vi "KlingerV2 Control.vi"(7 "Axe":u8(ring)=3 items=["W", "X", "Y", "Z"], 8 "error in":errorcluster, 9 "PosDem":dbl caption="Allez à" min=-79999.999 max=79999.999 step=0.001 format="%.3f", 10 "Relatif":bool caption="Relatif/Absolu\n(Absolu)", 11 "VISA Rsrc":refnum<visa-resource-name>="SR530") -> (0 "error out":errorcluster, 1 "Position":dbl min=-79999.999 max=79999.999 step=0.001 format="%.3f", 2 "NLimit":bool caption="Limite -", 3 "PLimit":bool caption="Limite +", 5 "Axe out":u8(ring)=3 caption="Axe" items=["W", "X", "Y", "Z"])   [LabVIEW 2019]
doc: "Ce Vi est une interface de contrôle complète d'où on peut effectué les diverse fonction du contrôlleur Klinger"
uses:
  <vilib>/Utility/error.llb/DialogType.ctl
  <userlib>/KlingerV2/KlingerV2 Params.ctl
  <userlib>/KlingerV2/KlingerV2 ConvUnitArr.vi
panel:
  in  "Save Par":bool
  in  "WriteAcc":bool
  in  "WriteSpeed":bool
  in  "Enable":bool caption="Motor\nEnable"
  in  "ReadPos":bool
  in  "ModParam":bool
  out "Nom de l'axe":string
  out "CorrParams":T1={"CorrActive"=FALSE, "ErreurLim"=0.1, "NbrEssais"=3} caption="Paramètres de \ncorrection de position" {"NbrEssais" min=1 max=5 step=1; "ErreurLim" min=0.0 max=10.0 step=0.1 format="%#.1f"}
  in  "Unit":u8(ring) caption="Unité:" items=["Pas", "mm", "ps", "Degré (°)"]
  in  "Default":bool
  in  "Zero":bool
  in  "Accel":dbl=0.4000000059604645 caption="Accélération" min=0.10000000149011612 max=2.0 step=0.10000000149011612 format="%#.1f"
  in  "Speed Type":enum32{"Pas/Seconde", "ms/Pas"}(radio)
  in  "Vitesse":i32=800 min=32 max=4000 step=1 format="%#.0f"
  in  "Quitter":bool
  in  "RAZ":bool
  in  "Origine":bool
  out "PosErreur":dbl caption="Erreur de\nPositionnement" min=-79999.999 max=79999.999 step=0.001 format="%.3f"
  out "Indcomm":string caption="Terminal Indicateur"
  out "Pos Init":dbl caption="Position Initiale" min=-79999.999 max=79999.999 step=0.001 format="%.3f"
  out "Moving":bool caption="Déplacement\nen cours"
  out "Erreur":bool
  # "Commandes"
  # "Paramètres"
  # "Sec"
  # "Relatif"
  # "Absolu"
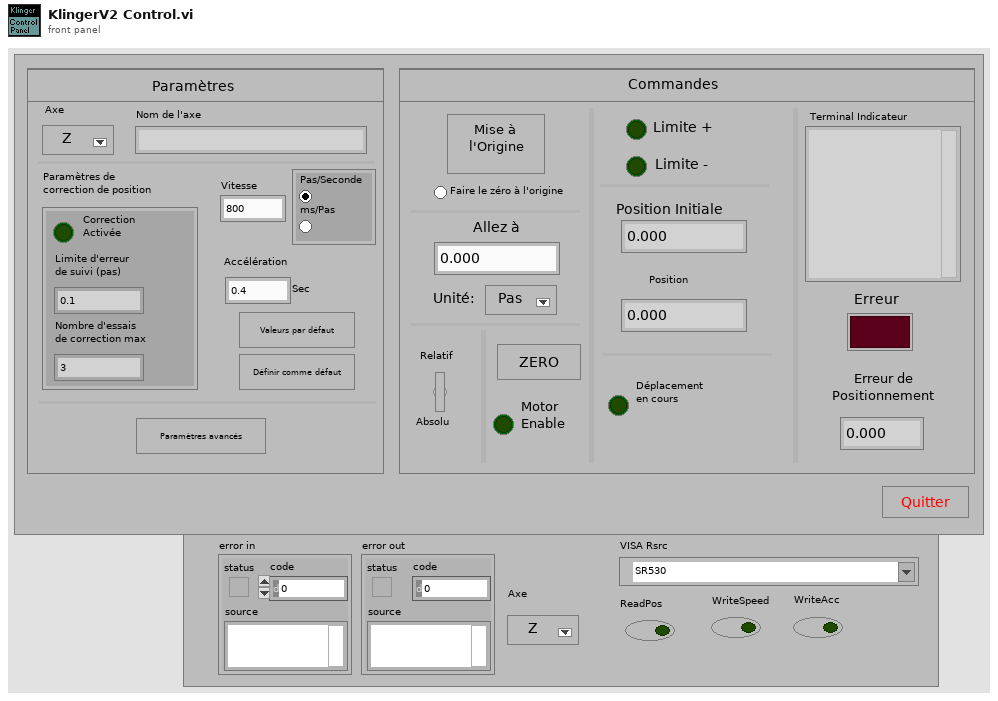
[diagram p1: front panel]
types:
  T1 = cluster{"CorrActive":bool, "ErreurLim":dbl, "NbrEssais":i32}
  T2 = cluster{"Position Ref":refnum<vi>, "Moving Ref":refnum<vi>, "PLimRef":refnum<vi>, "NLimRef":refnum<vi>}
  T3 = typedef "KlingerV2 Params.ctl" = enum16{"Type", "Origine", "Encodeur", "TypeMouv", "FactConv", "Nom", "CorrParams", "KlingCtrlPar", "Speed", "Acc", "Avance", "Tous"}
  T4 = cluster{"Minimum":dbl, "Maximum":dbl, "Increment":dbl}
  T5 = typedef "DialogType.ctl" = u16
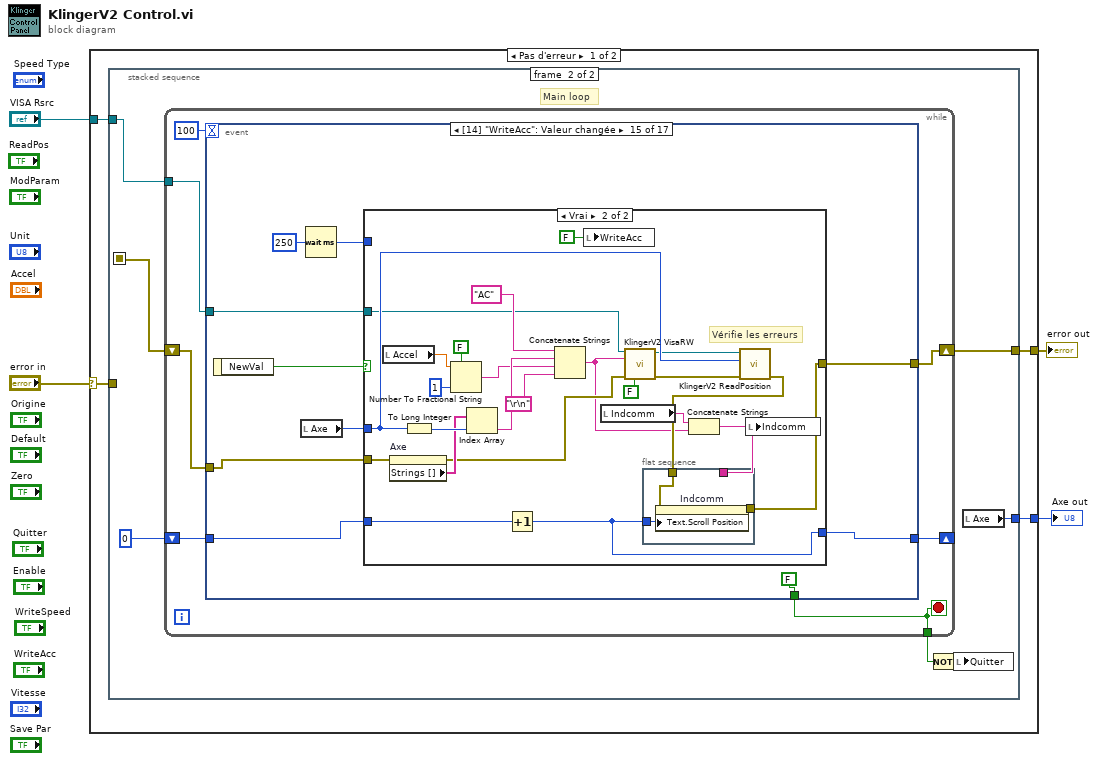
[diagram p0: block diagram]
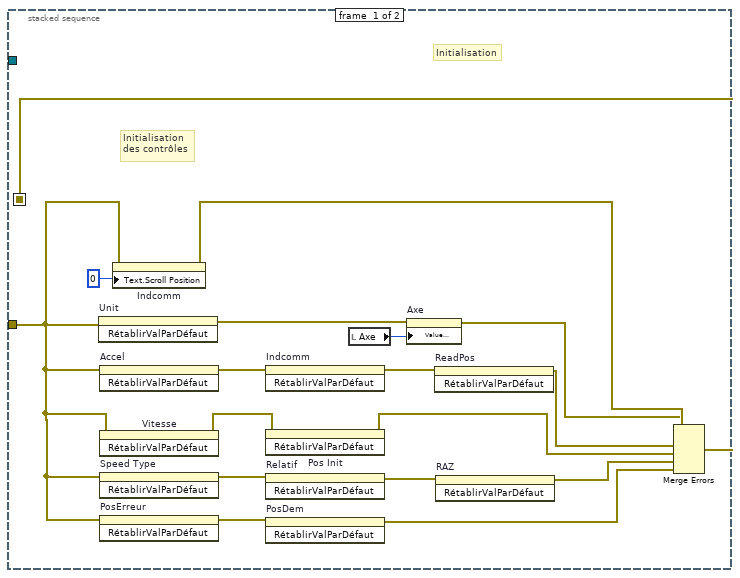
[diagram p2: hidden frame]
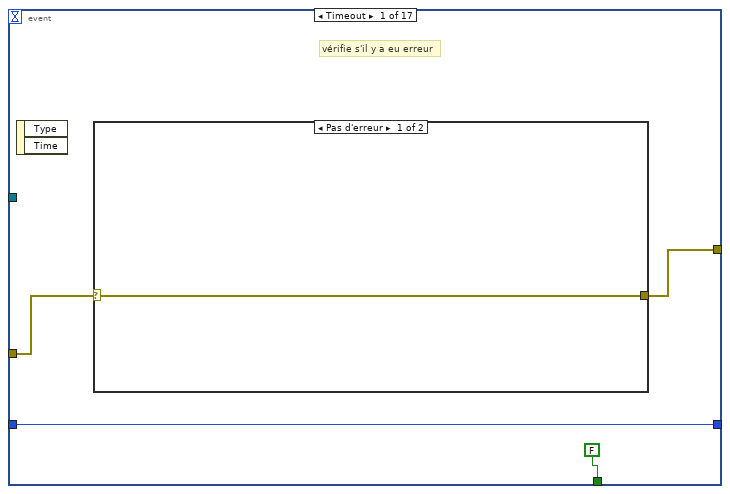
[diagram p3: hidden frame]
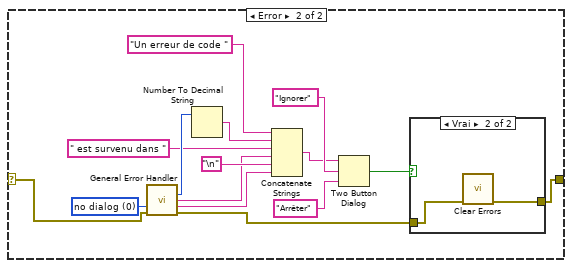
[diagram p4: hidden frame]
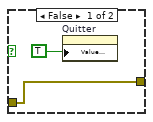
[diagram p5: hidden frame]
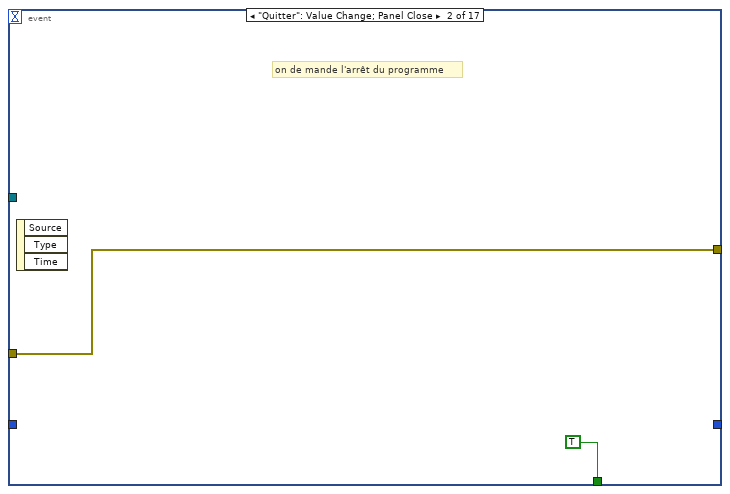
[diagram p6: hidden frame]
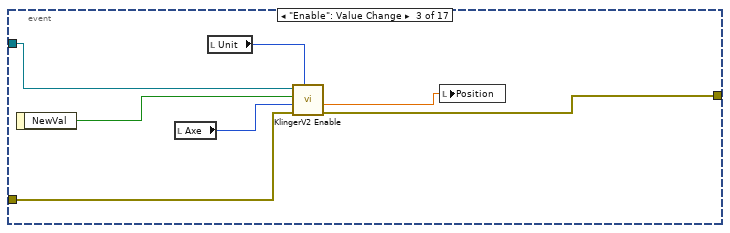
[diagram p7: hidden frame]
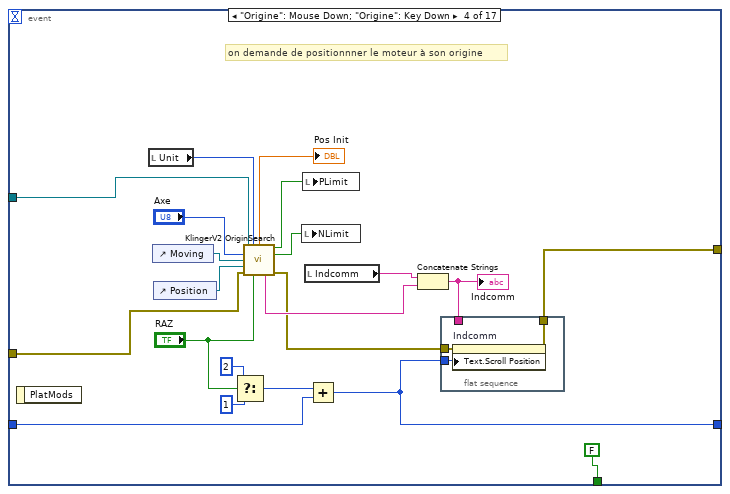
[diagram p8: hidden frame]
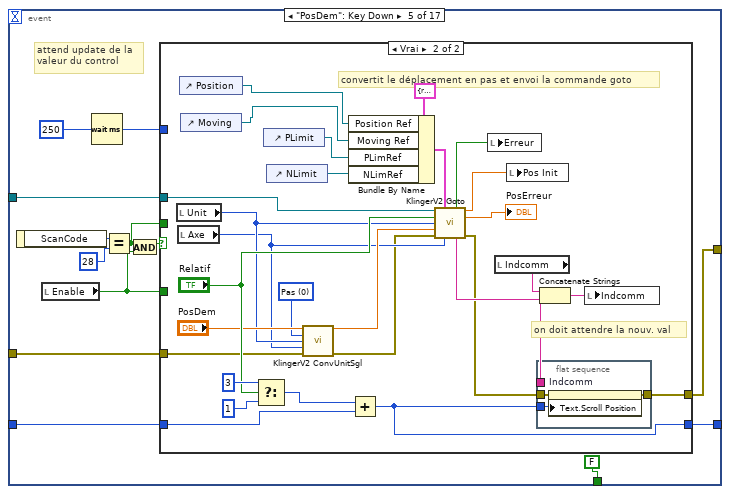
[diagram p9: hidden frame]
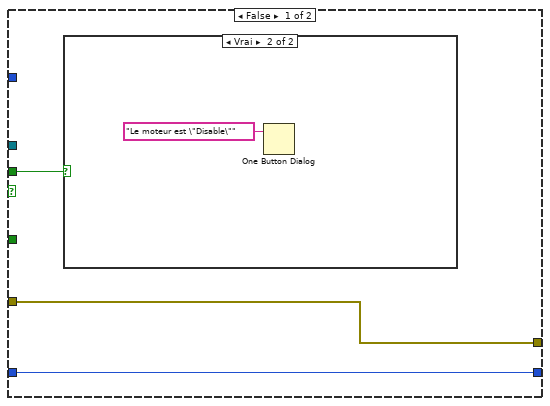
[diagram p10: hidden frame]
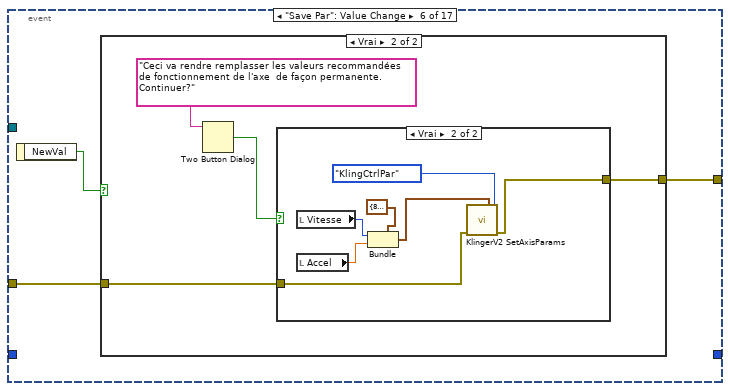
[diagram p12: hidden frame]
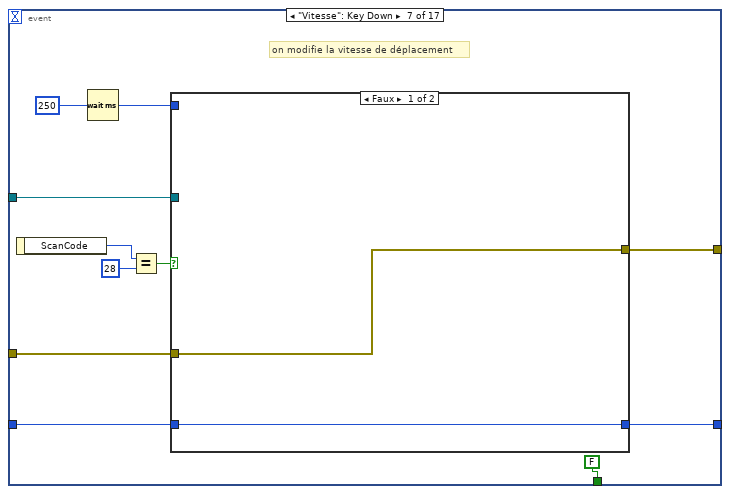
[diagram p15: hidden frame]
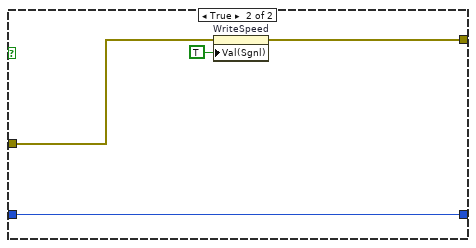
[diagram p16: hidden frame]
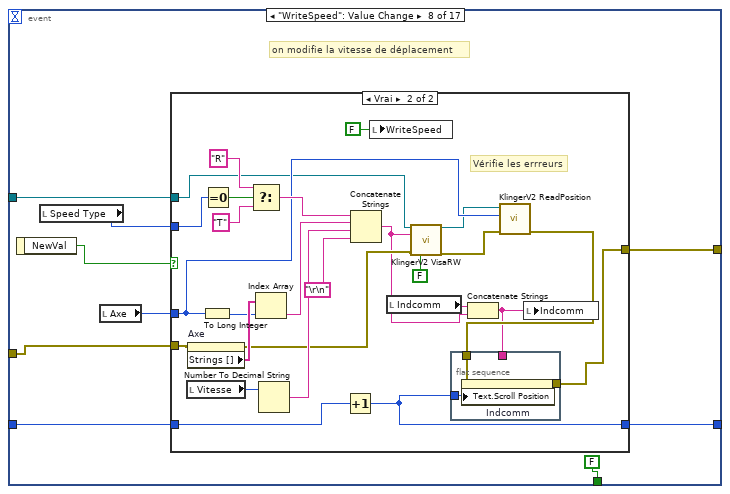
[diagram p17: hidden frame]
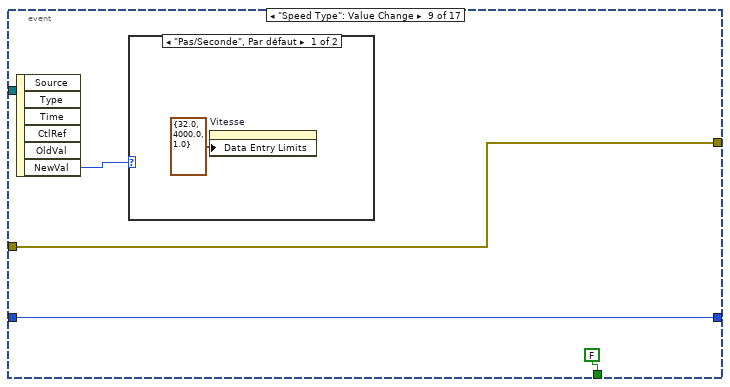
[diagram p19: hidden frame]
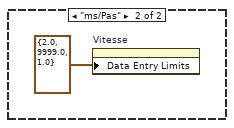
[diagram p20: hidden frame]
diagram:
  n1 = case shown="Pas d'erreur" "error in" {
    selector: "error in" -> [w7 w405]
    tunnel: [w8 w405] -> w4
    tunnel: [w6 u8 0 ("Axe")] -> w2
    tunnel: "VISA Rsrc" -> [w5 _]
    frame No Error {
      n2 = stacked-sequence {
        seq-local: [w16 _] -> [_ w31]
        tunnel: [_ w32] -> w8
        tunnel: w7 -> [w19 _]
        tunnel: [_ w27] -> w6
        tunnel: w5 -> [_ w26]
        frame #0 {
          # "Initialisation\ndes contrôles"
          # "Initialisation"
          n3 = invoke on="Unit" class="Ring (strict)" method="RétablirValParDéfaut"(error in=w19) -> (error out=w17:errorcluster)  [unwired: 2 in, 2 out]
          n4 = invoke on="Accel" class="NumDig (strict)" method="RétablirValParDéfaut"(error in=w19) -> (error out=w24:errorcluster)  [unwired: 2 in, 2 out]
          n5 = invoke on="Vitesse" class="DigNum (strict)" method="RétablirValParDéfaut"(error in=w19) -> (error out=w23:errorcluster)  [unwired: 2 in, 2 out]
          n6 = invoke on="Speed Type" class="RadioBtnsControl (strict)" method="RétablirValParDéfaut"(error in=w19) -> (error out=w22:errorcluster)  [unwired: 2 in, 2 out]
          n7 = invoke on="PosErreur" class="DigNum (strict)" method="RétablirValParDéfaut"(error in=w19) -> (error out=w21:errorcluster)  [unwired: 2 in, 2 out]
          n8 = property on="Indcomm" class="Ch"(error in=w19, "Text.Scroll Position"=u32 0) -> (error out=w15:errorcluster)  [unwired: 1 in, 1 out]
          n9 = invoke on="Indcomm" class="Str" method="RétablirValParDéfaut"(error in=w24) -> (error out=w18:errorcluster)  [unwired: 2 in, 2 out]
          n10 = invoke on="Pos Init" class="DigNum (strict)" method="RétablirValParDéfaut"(error in=w23) -> (error out=w12:errorcluster)  [unwired: 2 in, 2 out]
          n11 = invoke on="Relatif" class="Bool (strict)" method="RétablirValParDéfaut"(error in=w22) -> (error out=w20:errorcluster)  [unwired: 2 in, 2 out]
          n12 = invoke on="PosDem" class="DigNum (strict)" method="RétablirValParDéfaut"(error in=w21) -> (error out=w10:errorcluster)  [unwired: 2 in, 2 out]
          n13 = local read "Axe"() -> (w9:u8)
          n14 = property on="Axe" class="MDér (strict)"(error in=w17, "Value (Signaling)"=w9) -> (error out=w14:errorcluster)  [unwired: 1 in, 1 out]
          n15 = invoke on="ReadPos" class="Boolean (strict)" method="RétablirValParDéfaut"(error in=w18) -> (error out=w13:errorcluster)  [unwired: 2 in, 2 out]
          n16 = invoke on="RAZ" class="Bool (strict)" method="RétablirValParDéfaut"(error in=w20) -> (error out=w11:errorcluster)  [unwired: 2 in, 2 out]
          n17 = Merge Errors(w15, w14, w13, w12, w11, w10) -> (w16:errorcluster)
        }
        frame #1 {
          # "Main loop"
          n18 = while {
            shift-right: [w35] -> w32
            shift-left: w31 -> [w38]
            shift-right: [w36] -> _
            shift-left: u32 0 ("Text.Scroll Position") -> [w37]
            tunnel: [w34] -> w29
            tunnel: w26 -> [w33]
            stop <- w34 stop-if-true
            n19 = event shown="[14] \"WriteAcc\": Valeur changée" {
              selector: _ -> [_ _ _ _ _ _ _ _ _ _ _ _ _ _ _ _ _]
              dyn-events: _ -> [_ _ _ _ _ _ _ _ _ _ _ _ _ _ _ _ _]
              timeout: 100 -> [_ _ _ _ _ _ _ _ _ _ _ _ _ _ _ _ _]
              tunnel: w38 -> [w40 w64 w68 w85 w108 w146 w169 w185 w220 w236 w263 w303 w326 w335 w352 w393 w401]
              tunnel: [w42 w64 w69 w81 w100 w145 w165 w182 w220 w245 w275 w302 w318 w332 w350 w387 w400] -> w35
              tunnel: w37 -> [w43 _ _ w90 w107 _ w168 w184 w219 _ _ _ _ w331 w349 w392 w399]
              tunnel: [w43 _ _ w89 w106 _ w167 w183 w219 _ _ _ _ w334 w351 w391 w399] -> w36
              tunnel: [FALSE TRUE _ FALSE FALSE _ FALSE FALSE FALSE FALSE _ _ _ FALSE FALSE FALSE FALSE] -> w34
              tunnel: w33 -> [_ _ w70 w73 w101 _ w161 w180 _ _ _ w301 _ w327 w345 w383 _]
              event Timeout {
                # "vérifie s'il y a eu erreur"
                n20 = event-data() -> ()  [unwired: 1 in, 2 out]
                n21 = case shown="Pas d'erreur" w40 {
                  selector: w40 -> [w44 w45]
                  tunnel: [w44 w46] -> w42
                  frame No Error {
                  }
                  frame Error {
                    w56 = T5 0 items=["no dialog", "OK message", "continue or stop message", "OK message + warnings", "continue/stop + warnings"] ("type of dialog (OK msg:1)")
                    n22 = call <vilib>:"General Error Handler.vi"("type of dialog (OK msg:1)"=w56, "error in (no error)"=w45) -> ("code out"=w52:i32, "source out"=w51:string, "message"=w49:string, "error out"=w47:errorcluster)  [unwired: 9 in, 1 out]
                    n23 = Number To Decimal String(number=w52) -> (decimal integer string=w53:string)  [unwired: 1 in]
                    n24 = Concatenate Strings("Un erreur de code " ("string"), w53, " est survenu dans " ("string"), w51, "\n", w49) -> (w48:string)
                    n25 = Two Button Dialog(message=w48, 1:"Arrêter" ("F button name (\"Cancel\")"), 2:"Ignorer" ("T button name (\"OK\")")) -> (T button?=w59:bool)
                    n26 = case shown="Vrai" w59 {
                      tunnel: w47 -> [w61 w63]
                      tunnel: [w61 w62] -> w46
                      frame False {
                        n27 = property on="Quitter" class="Bool (strict)"("Value (Signaling)"=TRUE) -> ()  [unwired: 2 in, 2 out]
                      }
                      frame True {
                        n28 = call <vilib>:"Clear Errors.vi"("error in (no error)"=w63) -> ("error out"=w62:errorcluster)  [unwired: 5 in, 1 out]
                      }
                    }
                  }
                }
              }
              event "Quitter": Value Change; Panel Close {
                # "on de mande l'arrêt du programme"
                n29 = event-data() -> ()  [unwired: 1 in, 3 out]
              }
              event "Enable": Value Change {
                n30 = event-data() -> ("NewVal"=w72:bool)  [unwired: 1 in]
                n31 = local read "Axe"() -> (w71:u8)
                n32 = local read "Unit"() -> (w67:u8)
                n33 = call <userlib>:"KlingerV2 Enable.vi"("UnitDem"=w67, "error in"=w68, "Axe"=w71, "Enable"=w72, "VISA Rsrc"=w70) -> ("error out"=w69:errorcluster, "Position"=w66:dbl)  [unwired: 2 out]
                n34 = local write "Position"(w66) -> ()
              }
              event "Origine": Mouse Down; "Origine": Key Down {
                # "on demande de positionnner le moteur à son origine"
                n35 = event-data() -> ()  [unwired: 1 in, 1 out]
                n36 = local read "Unit"() -> (w76:u8)
                n37 = control-ref of="Moving"() -> (w75:refnum<vi>)
                n38 = control-ref of="Position"() -> (w91:refnum<vi>)
                n39 = Select(t=u32 2 ("x+y"), s="RAZ", f=u32 1 ("x+y")) -> (s? t:f=w88:u32)
                n40 = call <userlib>:"KlingerV2 OriginSearch.vi"("VISA Rsrc"=w73, "UnitDem"=w76, "Axe"="Axe", "Moving Ref"=w75, "Position Ref"=w91, "error in"=w85, "Set as Zero"="RAZ") -> ("Pos Init"=→"Pos Init":dbl, "PLimit"=w92:bool, "NLimit"=w93:bool, "Indcomm"=w83:string, "error out"=w82:errorcluster)  [unwired: 2 in, 2 out]
                n41 = local write "NLimit"(w93) -> ()
                n42 = local write "PLimit"(w92) -> ()
                n43 = local read "Indcomm"() -> (w84:string)
                n44 = Add(x=w88, y=w90) -> (x+y=w89:u32)
                n45 = Concatenate Strings(w84, w83) -> (w78:string)
                "Indcomm" <- w78
                n46 = flat-sequence {
                  tunnel: w89 -> [w96]
                  tunnel: w78 -> [_]
                  tunnel: w82 -> [w95]
                  tunnel: [w94] -> w81
                  frame #0 {
                    n47 = property on="Indcomm" class="Ch"(error in=w95, "Text.Scroll Position"=w96) -> (error out=w94:errorcluster)  [unwired: 1 in, 1 out]
                  }
                }
              }
              event "PosDem": Key Down {
                # "attend update de la \nvaleur du control"
                n48 = event-data() -> ("ScanCode"=w105:i16)  [unwired: 1 in]
                n49 = local read "Enable"() -> (w98:bool)
                n50 = Wait (ms)(milliseconds to wait=u32 250) -> (millisecond timer value=w103:u32)
                n51 = Equal?(x=w105, y=i16 28) -> (x = y?=w97:bool)
                n52 = And(x=w97, y=w98) -> (x .and. y?=w99:bool)
                n53 = case shown="Vrai" w99 {
                  tunnel: w108 -> [w111 w125]
                  tunnel: w107 -> [w112 w141]
                  tunnel: [w112 w134] -> w106
                  tunnel: w103 -> [_ _]
                  tunnel: w101 -> [_ w123]
                  tunnel: [w111 w135] -> w100
                  tunnel: w98 -> [_ _]
                  tunnel: w97 -> [w110 _]
                  frame False {
                    n54 = case shown="Vrai" w110 {
                      frame False {
                      }
                      frame True {
                        n55 = One Button Dialog(message="Le moteur est \"Disable\"") -> ()  [unwired: 1 in, 1 out]
                      }
                    }
                  }
                  frame True {
                    w129 = u8 0 items=["Pas", "mm", "ps"] ("UnitDem")
                    # "convertit le déplacement en pas et envoi la commande goto"
                    # "on doit attendre la nouv. val"
                    n56 = local read "Unit"() -> (w127:u8)
                    n57 = local read "Axe"() -> (w126:u8)
                    n58 = control-ref of="Position"() -> (w117:refnum<vi>)
                    n59 = control-ref of="Moving"() -> (w118:refnum<vi>)
                    n60 = Select(t=u32 3 ("Text.Scroll Position"), s="Relatif", f=u32 1 ("Text.Scroll Position")) -> (s? t:f=w138:u32)
                    n61 = control-ref of="PLimit"() -> (w116:refnum<vi>)
                    n62 = control-ref of="NLimit"() -> (w115:refnum<vi>)
                    n63 = call <userlib>:"KlingerV2 ConvUnitSgl.vi"("ParamAct"="PosDem", "UnitDem"=w129, "UnitAct"=w127, "Axe"=w126, "error in"=w125) -> ("ParamDem"=w128:dbl, "error out"=w124:errorcluster)  [unwired: 9 in]
                    n64 = Bundle By Name(cluster=T2 {"Position Ref"=refnum, "Moving Ref"=refnum, "PLimRef"=refnum, "NLimRef"=refnum} ("Ctrl Refs"), "Position Ref"=w117, "Moving Ref"=w118, "PLimRef"=w116, "NLimRef"=w115) -> (w120:T2)
                    n65 = Add(x=w138, y=w141) -> (x+y=w134:u32)
                    n66 = call <userlib>:"KlingerV2 Goto.vi"("VISA Rsrc"=w123, "Ctrl Refs"=w120, "Relatif"="Relatif", "UnitDem"=w127, "PosDem"=w128, "error in"=w124, "Axe"=w126) -> ("Erreur"=w114:bool, "Pos Init"=w119:dbl, "PosErreur"=→"PosErreur":dbl, "Indcomm"=w136:string, "error out"=w131:errorcluster)  [unwired: 2 in, 2 out]
                    n67 = local write "Erreur"(w114) -> ()
                    n68 = local read "Indcomm"() -> (w137:string)
                    n69 = local write "Pos Init"(w119) -> ()
                    n70 = flat-sequence {
                      tunnel: w134 -> [w144]
                      tunnel: w131 -> [w143]
                      tunnel: [w142] -> w135
                      tunnel: w133 -> [_]
                      frame #0 {
                        n71 = property on="Indcomm" class="Ch"(error in=w143, "Text.Scroll Position"=w144) -> (error out=w142:errorcluster)  [unwired: 1 in, 1 out]
                      }
                    }
                    n72 = Concatenate Strings(w137, w136) -> (w133:string)
                    n73 = local write "Indcomm"(w133) -> ()
                  }
                }
              }
              event "Save Par": Value Change {
                n74 = event-data() -> ("NewVal"=w147:bool)  [unwired: 1 in]
                n75 = case shown="Vrai" w147 {
                  tunnel: w146 -> [w148 w150]
                  tunnel: [w148 w149] -> w145
                  frame False {
                  }
                  frame True {
                    n76 = Two Button Dialog(message="Ceci va rendre remplasser les valeurs recommandées de fonctionnement de l'axe  de façon permanente. Continuer?") -> (T button?=w151:bool)  [unwired: 2 in]
                    n77 = case shown="Vrai" w151 {
                      tunnel: w150 -> [w153 w157]
                      tunnel: [w153 w156] -> w149
                      frame False {
                      }
                      frame True {
                        n78 = local read "Vitesse"() -> (w155:i32)
                        n79 = local read "Accel"() -> (w154:dbl)
                        n80 = Bundle(cluster=cluster{"Vitesse":i32, "Accel":dbl} {"Vitesse"=800, "Accel"=0.4000000059604645} ("Speed"), "Vitesse"=w155, "Accel"=w154) -> (w159:cluster{"Vitesse":i32, "Accel":dbl})
                        n81 = call <userlib>:"KlingerV2 SetAxisParams.vi"("Speed"=w159, "Param"=KlingerV2_Params."KlingCtrlPar", "error in"=w157) -> ("error out"=w156:errorcluster)  [unwired: 12 in]
                      }
                    }
                  }
                }
              }
              event "Vitesse": Key Down {
                # "on modifie la vitesse de déplacement"
                n82 = event-data() -> ("ScanCode"=w166:i16)  [unwired: 1 in]
                n83 = Wait (ms)(milliseconds to wait=u32 250) -> (millisecond timer value=w162:u32)
                n84 = Equal?(x=w166, y=i16 28) -> (x = y?=w170:bool)
                n85 = case shown="Faux" w170 {
                  tunnel: [w173 w175] -> w165
                  tunnel: w169 -> [w173 w174]
                  tunnel: w168 -> [w172 w177]
                  tunnel: [w172 w177] -> w167
                  tunnel: w162 -> [_ _]
                  tunnel: w161 -> [_ _]
                  frame False {
                  }
                  frame True {
                    n86 = property on="WriteSpeed" class="Bool (strict)"(error in=w174, "Val(Sgnl)"=TRUE ("Valeur (Signalisation)")) -> (error out=w175:errorcluster)  [unwired: 1 in, 1 out]
                  }
                }
              }
              event "WriteSpeed": Value Change {
                # "on modifie la vitesse de déplacement"
                n87 = event-data() -> ("NewVal"=w178:bool)  [unwired: 1 in]
                n88 = local read "Speed Type"() -> (w179:enum32{"Pas/Seconde", "ms/Pas"})
                n89 = local read "Axe"() -> (w186:u8)
                n90 = case shown="Vrai" w178 {
                  tunnel: w179 -> [_ w213]
                  tunnel: w186 -> [_ w201]
                  tunnel: [w188 w199] -> w182
                  tunnel: w185 -> [w188 w203]
                  tunnel: w184 -> [w187 w198]
                  tunnel: [w187 w202] -> w183
                  tunnel: w180 -> [_ w193]
                  frame False {
                  }
                  frame True {
                    # "Vérifie les errreurs"
                    n91 = local read "Vitesse"() -> (w189:i32)
                    n92 = property on="Axe" class="MDér (strict)"(error in=w203) -> (error out=w196:errorcluster, "Strings []"=w209:string[])  [unwired: 1 in, 1 out]
                    n93 = To Long Integer(number=w201) -> (32bit integer=w208:i32)
                    n94 = Equal To 0?(x=w213) -> (x = 0?=w212:bool)
                    n95 = Select(t="R", s=w212, f="T") -> (s? t:f=w210:string)
                    n96 = Index Array(array=w209, index=w208) -> (element=w207:string)
                    n97 = Number To Decimal String(number=w189) -> (decimal integer string=w205:string)  [unwired: 1 in]
                    n98 = Increment(x=w198) -> (x+1=w202:u32)
                    n99 = Concatenate Strings(w210, w207, w205, "\r\n") -> (w194:string)
                    n100 = local write "WriteSpeed"(FALSE ("WriteSpeed")) -> ()
                    n101 = local read "Indcomm"() -> (w204:string)
                    n102 = call <userlib>:"KlingerV2 VisaRW.vi"("VISA Rsrc"=w193, "ChaineCom"=w194, "error in (no error)"=w196, "Lecture?(T)"=FALSE) -> ("VISA Rsrc Out"=w191:refnum<visa-resource-name>, "error out"=w195:errorcluster)  [unwired: 7 in, 3 out]
                    n103 = flat-sequence {
                      tunnel: w202 -> [w217]
                      tunnel: w200 -> [w216]
                      tunnel: [w215] -> w199
                      tunnel: w197 -> [_]
                      frame #0 {
                        n104 = property on="Indcomm" class="Ch"(error in=w216, "Text.Scroll Position"=w217) -> (error out=w215:errorcluster)  [unwired: 1 in, 1 out]
                      }
                    }
                    n105 = Concatenate Strings(w204, w194) -> (w197:string)
                    n106 = call <userlib>:"KlingerV2 ReadPosition.vi"("error in"=w195, "Axe"=w201, "VISA Rsrc"=w191) -> ("error out"=w200:errorcluster)  [unwired: 2 in, 6 out]
                    n107 = local write "Indcomm"(w197) -> ()
                  }
                }
              }
              event "Speed Type": Value Change {
                n108 = event-data() -> ("NewVal"=w221:enum32{"Pas/Seconde", "ms/Pas"})  [unwired: 1 in, 5 out]
                n109 = case shown="\"Pas/Seconde\", Par défaut" w221 {
                  frame "Pas/Seconde", Default {
                    n110 = property on="Vitesse" class="NumNb (strict)"("Data Entry Limits"=T4 {"Minimum"=32.0, "Maximum"=4000.0, "Increment"=1.0} ("Data Range")) -> ()  [unwired: 2 in, 2 out]
                  }
                  frame "ms/Pas" {
                    n111 = property on="Vitesse" class="NumNb (strict)"("Data Entry Limits"=T4 {"Minimum"=2.0, "Maximum"=9999.0, "Increment"=1.0} ("Data Range")) -> ()  [unwired: 2 in, 2 out]
                  }
                }
              }
              event "Unit": Value Change {
                # "convertit les valeurs des contrôles"
                # "en fonction de l'unité choisi"
                # "et Modifie la précision des indic."
                # "Modifie le range des indic."
                n112 = event-data() -> ("NewVal"=w226:u8, "OldVal"=w224:u8)  [unwired: 1 in]
                n113 = local read "Position"() -> (w249:dbl)
                n114 = local read "PosDem"() -> (w250:dbl)
                n115 = local read "PosErreur"() -> (w251:dbl)
                n116 = local read "Pos Init"() -> (w248:dbl)
                n117 = local read "Axe"() -> (w225:u8)
                n118 = call <userlib>:"KlingerV2 ControlLimit.vi"("Axe"=w225, "UnitDem"=w226, "error in"=w236) -> ("DataRange"=w234:T4, "FormtPrec"=w233:cluster{"Format":u8, "Precision":u8}, "error out"=w235:errorcluster)  [unwired: 2 in]
                n119 = Build Array(w249, w250, w251, w248) -> (w243:dbl[])
                n120 = property on="Position" class="NumNb (strict)"(error in=w235, "Data Entry Limits"=w234) -> (error out=w232:errorcluster)  [unwired: 1 in, 1 out]
                n121 = property on="PosErreur" class="NumNb (strict)"(error in=w235, "Data Entry Limits"=w234) -> (error out=w231:errorcluster)  [unwired: 1 in, 1 out]
                n122 = property on="Pos Init" class="NumNb (strict)"(error in=w232, "Data Entry Limits"=w234) -> (error out=w227:errorcluster)  [unwired: 1 in, 1 out]
                n123 = property on="PosDem" class="NumNb (strict)"(error in=w231, "Data Entry Limits"=w234) -> (error out=w228:errorcluster)  [unwired: 1 in, 1 out]
                n124 = call-poly <userlib>:"KlingerV2 ConvUnit.vi"("ParamAct"=w243, "UnitDem"=w226, "UnitAct"=w224, "Axe"=w225, "error in"=w235) -> ("ParamDem"=w242:dbl[], "error out"=w237:errorcluster)  [unwired: 9 in]
                n125 = property on="Position" class="NumNb (strict)"(error in=w227, "Display Format"=w233) -> (error out=w230:errorcluster)  [unwired: 1 in, 1 out]
                n126 = property on="PosErreur" class="NumNb (strict)"(error in=w228, "Display Format"=w233) -> (error out=w229:errorcluster)  [unwired: 1 in, 1 out]
                n127 = property on="Pos Init" class="NumNb (strict)"(error in=w230, "Display Format"=w233) -> (error out=w247:errorcluster)  [unwired: 1 in, 1 out]
                n128 = property on="PosDem" class="NumNb (strict)"(error in=w229, "Display Format"=w233) -> (error out=w246:errorcluster)  [unwired: 1 in, 1 out]
                n129 = Index Array(array=w242) -> (element #1=w241:dbl, element #2=w240:dbl, element #3=w239:dbl, element #4=w238:dbl)  [unwired: 4 in]
                n130 = Merge Errors(w247, w246, w237) -> (w245:errorcluster)
                n131 = local write "Position"(w241) -> ()
                n132 = local write "PosDem"(w240) -> ()
                n133 = local write "PosErreur"(w239) -> ()
                n134 = local write "Pos Init"(w238) -> ()
              }
              event "Axe": Value Change {
                w253 = TRUE ("Valeur (Signalisation)")
                w276 = u8 0 items=["Pas", "mm", "ps", "Degré (°)"] ("UnitDem")
                w289 = i32[] [1, 2]  # Rot Dis
                w290 = i32[] [3]  # Linear Dis
                w294 = u8 2  # Dis
                w293 = u8 0  # en
                w296 = u8 2  # Dis
                w297 = u8 0  # en
                # "Modifie la précision des indic."
                # "Modifie le range des indic."
                n135 = event-data() -> ("NewVal"=w268:u8)  [unwired: 1 in, 1 out]
                n136 = call <userlib>:"KlingerV2 GetAxisParams.vi"("Axe"=w268, "Param"=KlingerV2_Params."Tous", "error in"=w263) -> ("Speed"=w259:cluster{"Vitesse":i32, "Accel":dbl}, "TypeMouv"=w288:i32, "Nom de l'axe"=→"Nom de l'axe":string, "CorrParams"=→"CorrParams":T1, "Encodeur"=w295:bool, "Origine"=w292:bool, "error out"=w269:errorcluster)  [unwired: 3 in, 3 out]
                n137 = Equal To 0?(x=w288) -> (x = 0?=w287:bool)
                n138 = Select(t=w293, s=w292, f=w294) -> (s? t:f=w291:u8)
                n139 = Select(t=w297, s=w295, f=w296) -> (s? t:f=w298:u8)
                n140 = property on="RAZ" class="Bool (strict)"(error in=w263, "Disabled"=w291) -> (error out=w274:errorcluster)  [unwired: 1 in, 1 out]
                n141 = property on="CorrParams" class="Clust (strict)"(error in=w263, "Disabled"=w298) -> (error out=w273:errorcluster)  [unwired: 1 in, 1 out]
                n142 = Select(t=w290, s=w287, f=w289) -> (s? t:f=w286:i32[])
                n143 = call <userlib>:"KlingerV2 ControlLimit.vi"("Axe"=w268, "UnitDem"=w276, "error in"=w263) -> ("DataRange"=w285:T4, "FormtPrec"=w284:cluster{"Format":u8, "Precision":u8}, "error out"=w277:errorcluster)  [unwired: 2 in]
                n144 = property on="Unit" class="MDér (strict)"(error in=w269, "Disabled Items []"=w286) -> (error out=w261:errorcluster)  [unwired: 1 in, 1 out]
                n145 = Unbundle By Name(w259) -> ("Vitesse"=w256:i32, "Accel"=w255:dbl)
                n146 = property on="Position" class="NumNb (strict)"(error in=w277, "Data Entry Limits"=w285) -> (error out=w283:errorcluster)  [unwired: 1 in, 1 out]
                n147 = property on="PosErreur" class="NumNb (strict)"(error in=w277, "Data Entry Limits"=w285) -> (error out=w282:errorcluster)  [unwired: 1 in, 1 out]
                n148 = local write "Vitesse"(w256) -> ()
                n149 = local write "Accel"(w255) -> ()
                n150 = property on="Speed Type" class="CmdeBtnsRadio (strict)"(error in=w261, "Value (Signaling)"=enum32{"Pas/Seconde", "ms/Pas"}."Pas/Seconde" ("Valeur (Signalisation)")) -> (error out=w258:errorcluster)  [unwired: 1 in, 1 out]
                n151 = Build Array(w274, w273) -> (w270:errorcluster[])
                n152 = property on="Pos Init" class="NumNb (strict)"(error in=w283, "Data Entry Limits"=w285) -> (error out=w278:errorcluster)  [unwired: 1 in, 1 out]
                n153 = property on="PosDem" class="NumNb (strict)"(error in=w282, "Data Entry Limits"=w285) -> (error out=w279:errorcluster)  [unwired: 1 in, 1 out]
                n154 = property on="WriteSpeed" class="Bool (strict)"(error in=w258, "Value (Signaling)"=w253) -> (error out=w257:errorcluster)  [unwired: 1 in, 1 out]
                n155 = property on="Position" class="NumNb (strict)"(error in=w278, "Display Format"=w284) -> (error out=w281:errorcluster)  [unwired: 1 in, 1 out]
                n156 = property on="PosErreur" class="NumNb (strict)"(error in=w279, "Display Format"=w284) -> (error out=w280:errorcluster)  [unwired: 1 in, 1 out]
                n157 = property on="WriteAcc" class="Bool (strict)"(error in=w257, "Value (Signaling)"=w253) -> (error out=w254:errorcluster)  [unwired: 1 in, 1 out]
                n158 = property on="Pos Init" class="NumNb (strict)"(error in=w281, "Display Format"=w284) -> (error out=w271:errorcluster)  [unwired: 1 in, 1 out]
                n159 = property on="PosDem" class="NumNb (strict)"(error in=w280, "Display Format"=w284) -> (error out=w272:errorcluster)  [unwired: 1 in, 1 out]
                n160 = property on="Enable" class="Bool (strict)"(error in=w254, "Value (Signaling)"=w253) -> (error out=w252:errorcluster)  [unwired: 1 in, 1 out]
                n161 = property on="Unit" class="MDér (strict)"(error in=w252, "Value (Signaling)"=u8 0) -> (error out=w266:errorcluster)  [unwired: 1 in, 1 out]
                n162 = property on="ReadPos" class="Bool (strict)"(error in=w266, "Value (Signaling)"=TRUE) -> (error out=w264:errorcluster)  [unwired: 1 in, 1 out]
                n163 = Merge Errors(w264, w271, w272, w270) -> (w275:errorcluster)
              }
              event "ReadPos": Value Change {
                n164 = event-data() -> ("NewVal"=w304:bool)  [unwired: 1 in]
                n165 = case shown="Vrai" w304 {
                  tunnel: w303 -> [w305 w314]
                  tunnel: [w305 w313] -> w302
                  tunnel: w301 -> [_ w306]
                  frame False {
                  }
                  frame True {
                    w316 = u8 0 items=["Pas", "mm", "ps", "Degré (°)"] ("UnitDem")
                    # "lit la position/statut"
                    n166 = local read "Axe"() -> (w315:u8)
                    n167 = call <userlib>:"KlingerV2 ReadPosition.vi"("error in"=w314, "UnitDem"=w316, "Axe"=w315, "VISA Rsrc"=w306) -> ("error out"=w313:errorcluster, "Statut"=→"Erreur":bool, "Position"=→"Position":dbl, "NLimit"=→"NLimit":bool, "Moving"=→"Moving":bool, "PLimit"=→"PLimit":bool)  [unwired: 1 in, 1 out]
                    n168 = local write "ReadPos"(FALSE ("ReadPos")) -> ()
                  }
                }
              }
              event "ModParam": Key Up; "ModParam": Mouse Up {
                w321 = u8 2  # Dis
                w322 = u8 0  # en
                n169 = event-data() -> ()  [unwired: 1 in, 5 out]
                n170 = local read "Axe"() -> (w325:u8)
                n171 = call <userlib>:"KlingerV2 AxisParams.vi"("Axe"=w325, "error in"=w326) -> ("Encodeur Out"=w320:bool, "Nom Out"=w324:string, "CorrParams out"=w317:T1, "error out"=w319:errorcluster)  [unwired: 10 in]
                n172 = local write "Nom de l'axe"(w324) -> ()
                n173 = local write "CorrParams"(w317) -> ()
                n174 = Select(t=w322, s=w320, f=w321) -> (s? t:f=w323:u8)
                n175 = property on="CorrParams" class="Clust (strict)"(error in=w319, "Disabled"=w323) -> (error out=w318:errorcluster)  [unwired: 1 in, 1 out]
              }
              event "Accel": Key Down {
                n176 = event-data() -> ("ScanCode"=w333:i16)  [unwired: 1 in]
                n177 = Wait (ms)(milliseconds to wait=u32 250) -> (millisecond timer value=w329:u32)
                n178 = Equal?(x=w333, y=i16 28) -> (x = y?=w336:bool)
                n179 = case shown="Vrai" w336 {
                  tunnel: w335 -> [w338 w341]
                  tunnel: w331 -> [w339 w343]
                  tunnel: [w339 w343] -> w334
                  tunnel: [w338 w342] -> w332
                  tunnel: w329 -> [_ _]
                  tunnel: w327 -> [_ _]
                  frame False {
                  }
                  frame True {
                    n180 = property on="WriteAcc" class="Bool (strict)"(error in=w341, "Val(Sgnl)"=TRUE ("Valeur (Signalisation)")) -> (error out=w342:errorcluster)  [unwired: 1 in, 1 out]
                  }
                }
              }
              event "WriteAcc": Value Change {
                n181 = event-data() -> ("NewVal"=w344:bool)  [unwired: 1 in]
                n182 = local read "Axe"() -> (w353:u8)
                n183 = Wait (ms)(milliseconds to wait=u32 250) -> (millisecond timer value=w347:u32)
                n184 = case shown="Vrai" w344 {
                  tunnel: w353 -> [_ w369]
                  tunnel: w352 -> [w354 w372]
                  tunnel: w349 -> [w355 w368]
                  tunnel: [w355 w367] -> w351
                  tunnel: [w354 w365] -> w350
                  tunnel: w347 -> [_ _]
                  tunnel: w345 -> [_ w361]
                  frame False {
                  }
                  frame True {
                    # "Vérifie les erreurs"
                    n185 = local read "Accel"() -> (w360:dbl)
                    n186 = property on="Axe" class="MDér (strict)"(error in=w372) -> (error out=w362:errorcluster, "Strings []"=w375:string[])  [unwired: 1 in, 1 out]
                    n187 = To Long Integer(number=w369) -> (32bit integer=w378:i32)
                    n188 = Number To Fractional String(use system decimal point (T)=FALSE, number=w360, precision (6)=i16 1) -> (F-format string=w374:string)  [unwired: 1 in]
                    n189 = Index Array(array=w375, index=w378) -> (element=w377:string)
                    n190 = Increment(x=w368) -> (x+1=w367:u32)
                    n191 = Concatenate Strings("AC" ("string"), w377, w374, "\r\n") -> (w359:string)
                    n192 = local write "WriteAcc"(FALSE ("WriteAcc")) -> ()
                    n193 = local read "Indcomm"() -> (w371:string)
                    n194 = call <userlib>:"KlingerV2 VisaRW.vi"("VISA Rsrc"=w361, "ChaineCom"=w359, "error in (no error)"=w362, "Lecture?(T)"=FALSE) -> ("VISA Rsrc Out"=w357:refnum<visa-resource-name>, "error out"=w363:errorcluster)  [unwired: 7 in, 3 out]
                    n195 = flat-sequence {
                      tunnel: w367 -> [w382]
                      tunnel: w366 -> [_]
                      tunnel: [w381] -> w365
                      tunnel: w364 -> [w380]
                      frame #0 {
                        n196 = property on="Indcomm" class="Ch"(error in=w380, "Text.Scroll Position"=w382) -> (error out=w381:errorcluster)  [unwired: 1 in, 1 out]
                      }
                    }
                    n197 = Concatenate Strings(w371, w359) -> (w366:string)
                    n198 = call <userlib>:"KlingerV2 ReadPosition.vi"("error in"=w363, "Axe"=w369, "VISA Rsrc"=w357) -> ("error out"=w364:errorcluster)  [unwired: 2 in, 6 out]
                    n199 = local write "Indcomm"(w366) -> ()
                  }
                }
              }
              event "Zero": Mouse Down; "Zero": Key Down {
                n200 = event-data() -> ()  [unwired: 1 in, 1 out]
                n201 = local read "Unit"() -> (w384:u8)
                n202 = control-ref of="Position"() -> (w394:refnum<vi>)
                n203 = local read "Axe"() -> (w395:u8)
                n204 = call <userlib>:"KlingerV2 SetZero.vi"("VISA Rsrc"=w383, "Position Ref"=w394, "Axe"=w395, "error in"=w393, "UnitDem"=w384) -> ("Ind Comm"=w389:string, "error out"=w388:errorcluster)  [unwired: 1 out]
                n205 = Increment(x=w392) -> (x+1=w391:u32)
                n206 = local read "Indcomm"() -> (w390:string)
                n207 = flat-sequence {
                  tunnel: w391 -> [w398]
                  tunnel: w388 -> [w397]
                  tunnel: [w396] -> w387
                  tunnel: w386 -> [_]
                  frame #0 {
                    n208 = property on="Indcomm" class="Ch"(error in=w397, "Text.Scroll Position"=w398) -> (error out=w396:errorcluster)  [unwired: 1 in, 1 out]
                  }
                }
                n209 = Concatenate Strings(w390, w389) -> (w386:string)
                n210 = local write "Indcomm"(w386) -> ()
              }
              event "Default": Key Down; "Default": Mouse Down {
                # "Recharge les valeur du fichier ini"
                n211 = event-data() -> ()  [unwired: 1 in, 5 out]
                n212 = local read "Axe"() -> (w402:u8)
                n213 = property on="Axe" class="MDér (strict)"(error in=w401, "Val(Sgnl)"=w402) -> (error out=w400:errorcluster)  [unwired: 1 in, 1 out]
              }
            }
          }
          n214 = Not(x=w29) -> (.not. x?=w28:bool)
          n215 = local write "Quitter"(w28) -> ()
          n216 = local read "Axe"() -> (w27:u8)
        }
      }
    }
    frame Error {
    }
  }
  "error out" <- w4
  "Axe out" <- w2
